vi "txrx-test.vi"() -> ()   [LabVIEW 2013]
uses:
  <vilib>/Analysis/2dsp.llb/Complex FFT.vi
  <vilib>/Analysis/2dsp.llb/Real FFT.vi
  <instrlib>/niUSRP/niUSRP Fetch Rx Data (CDB).vi
  <instrlib>/niUSRP/niUSRP Write Tx Data (CDB).vi
  <vilib>/Analysis/NI_AALBase.lvlib
  <vilib>/Analysis/NI_AALPro.lvlib
panel:
  out "coerced gain 2":dbl format="%#_6f"
  out "coerced IQ rate 2":dbl=100000.0 format="%#_6p"
  out "input":dbl[](graph)
  out "output":dbl[](graph)
  in  "stop 2":bool
  out "coerced carrier frequency":dbl
  out "coerced IQ rate":dbl=100000.0 format="%#_6p"
  out "coerced gain":dbl format="%#_6f"
  in  "stop":bool
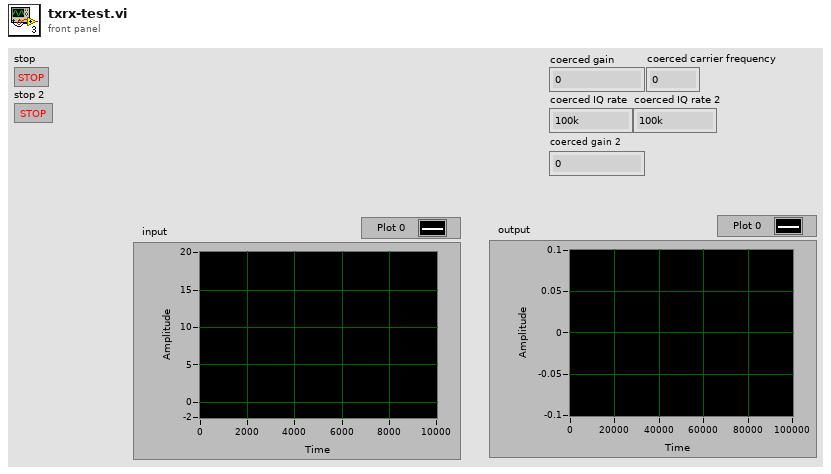
[diagram p1: front panel]
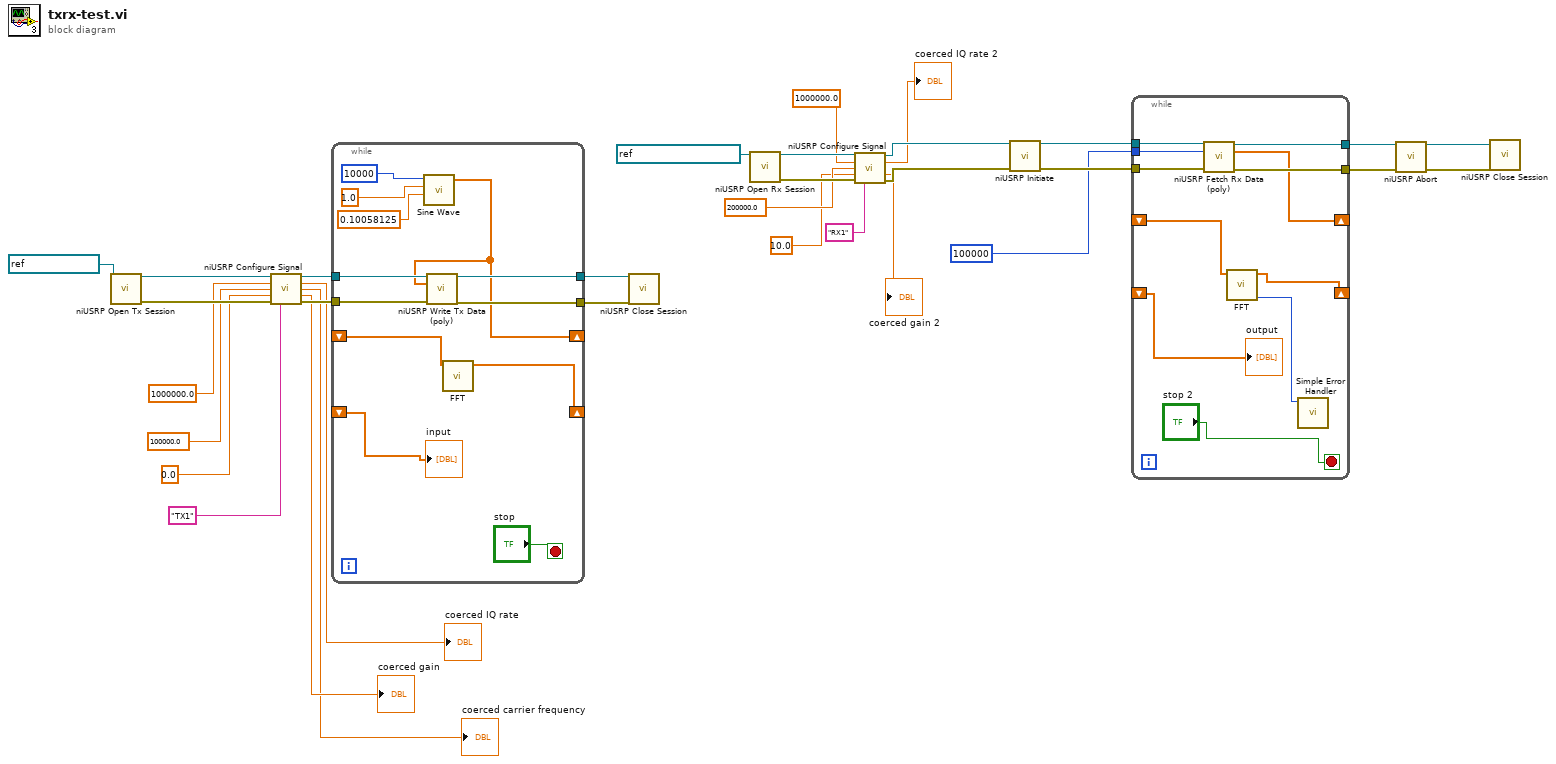
[diagram p0: block diagram]
diagram:
  n1 = call <instrlib>:"niUSRP Open Tx Session.vi"("device names"=refnum<k15> "192.168.10.8") -> ("session handle out"=w28:refnum<k15>, "error out"=w27:errorcluster)  [unwired: 13 in]
  n2 = call <instrlib>:"niUSRP Configure Signal.vi"("session handle"=w28, "IQ rate"=1000000.0, "carrier frequency"=100000.0, "gain"=0.0, "error in (no error)"=w27, "active antenna"="TX1") -> ("session handle out"=w32:refnum<k15>, "coerced IQ rate"=→"coerced IQ rate":dbl, "coerced carrier frequency"=→"coerced carrier frequency":dbl, "coerced gain"=→"coerced gain":dbl, "error out"=w31:errorcluster)  [unwired: 5 in]
  n3 = while {
    tunnel: w32 -> [w44]
    tunnel: w31 -> [w43]
    tunnel: [w42] -> w30
    tunnel: [w41] -> w29
    shift-right: [w36] -> _
    shift-left: _ -> [w35]
    shift-right: [w34] -> _
    shift-left: _ -> [w33]
    stop <- "stop" stop-if-true
    n4 = call <vilib>:"Sine Wave.vi"("samples"=10000, "amplitude"=1.0, "frequency"=0.10058125) -> ("sine wave"=w36:dbl[])  [unwired: 2 in, 2 out]
    n5 = call-poly <instrlib>:"niUSRP Write Tx Data (poly).vi"("session handle"=w44, "data"=w36, "error in (no error)"=w43) -> ("session handle out"=w42:refnum<k15>, "error out"=w41:errorcluster)  [unwired: 11 in]
    n6 = call-poly <vilib>:"FFT.vi"("X"=w35) -> ("FFT {X}"=w34:cdb[])  [unwired: 9 in, 1 out]
    "input" <- w33
  }
  n7 = call <instrlib>:"niUSRP Close Session.vi"("session handle"=w30, "error in (no error)"=w29) -> ()  [unwired: 13 in, 1 out]
  n8 = call <instrlib>:"niUSRP Open Rx Session.vi"("device names"=refnum<k15> "192.168.10.9") -> ("session handle out"=w18:refnum<k15>, "error out"=w17:errorcluster)  [unwired: 13 in]
  n9 = call <instrlib>:"niUSRP Configure Signal.vi"("session handle"=w18, "IQ rate"=1000000.0, "carrier frequency"=200000.0, "gain"=10.0, "error in (no error)"=w17, "active antenna"="RX1") -> ("session handle out"=w16:refnum<k15>, "coerced IQ rate"=→"coerced IQ rate 2":dbl, "coerced gain"=→"coerced gain 2":dbl, "error out"=w15:errorcluster)  [unwired: 5 in, 1 out]
  n10 = call <instrlib>:"niUSRP Initiate.vi"("session handle"=w16, "error in (no error)"=w15) -> ("session handle out"=w14:refnum<k15>, "error out"=w13:errorcluster)  [unwired: 12 in]
  n11 = while {
    tunnel: w14 -> [w55]
    tunnel: w13 -> [w54]
    tunnel: [w53] -> w12
    tunnel: [w52] -> w11
    tunnel: i64 100000 ("number of samples") -> [w51]
    shift-right: [w50] -> _
    shift-left: _ -> [w49]
    shift-right: [w48] -> _
    shift-left: _ -> [w47]
    stop <- "stop 2" stop-if-true
    n12 = call-poly <instrlib>:"niUSRP Fetch Rx Data (poly).vi"("session handle"=w55, "number of samples"=w51, "error in (no error)"=w54) -> ("session handle out"=w53:refnum<k15>, "data"=w50:cdb[], "error out"=w52:errorcluster)  [unwired: 9 in, 1 out]
    n13 = call-poly <vilib>:"FFT.vi"("X"=w49) -> ("error"=w46:i32, "FFT {X}"=w48:cdb[])  [unwired: 9 in]
    n14 = call <vilib>:"Simple Error Handler.vi"("error code (no error:0)"=w46) -> ()  [unwired: 4 in, 5 out]
    "output" <- w47
  }
  n15 = call <instrlib>:"niUSRP Abort.vi"("session handle"=w12, "error in (no error)"=w11) -> ("session handle out"=w10:refnum<k15>, "error out"=w9:errorcluster)  [unwired: 12 in]
  n16 = call <instrlib>:"niUSRP Close Session.vi"("session handle"=w10, "error in (no error)"=w9) -> ()  [unwired: 13 in, 1 out]
